vi "BSON_bytes_to_data_strict.vi"(7 "dataType":variant, 8 "error in (no error)":errorcluster, 11 "BSONbytes":u8[](array[numeric])) -> (0 "error out":errorcluster, 3 "result":variant)   [LabVIEW 2015, in "BSON_convertors_Library.lvlib"]
doc: "Converts the input byte stream into data fields and populates the input field with these values.\nNames, field types and their order must be the same in both structures"
uses:
  BSON_convertors_Library.lvlib
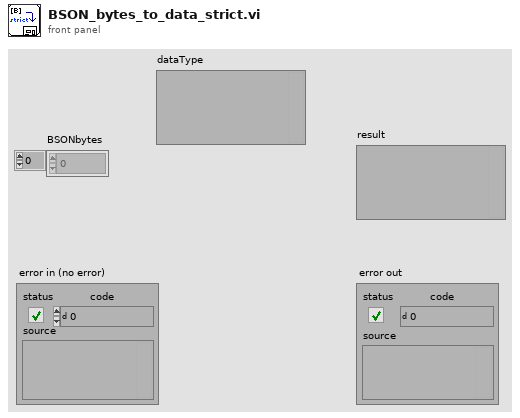
[diagram p1: front panel]
types:
  T1 = typedef "BSON_convertors_Library.lvlib/BSONelement.ctl" = cluster{"dataType":T2, "name":string, "value":variant}
  T2 = typedef "BSON_convertors_Library.lvlib/dataType.ctl" = enum8{"empty(terminator)", "double", "string", "document", "array", "binary", "Deprecated(Undefined)", "ObjectId", "boolean", "UTC datetime", "Null value", "cstring", "Deprecated(DBPointer)", "JavaScript", "Deprecated(Symbol)", "code_w_s", "int32", "uint64", "int64", "ext (decimal128)", "Min key", "Max key"}
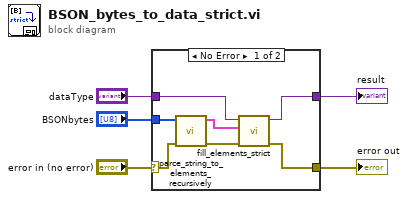
[diagram p0: block diagram]
diagram:
  n1 = case shown="No Error" "error in (no error)" {
    selector: "error in (no error)" -> [w11 w14]
    tunnel: "BSONbytes" -> [w12 _]
    tunnel: "dataType" -> [w10 w13]
    tunnel: [w6 w14] -> w2
    tunnel: [w7 w13] -> w1
    frame No Error {
      n2 = call "parce_string_to_elements_recursively.vi"("error in (no error)"=w11, "BSONdoc"=w12) -> ("error out"=w9:errorcluster, "arrayOfElements"=w8:T1[])  [unwired: 8 in]
      n3 = call "fill_elements_strict.vi"("error in (no error)"=w9, "arrayOfElements"=w8, "dataType in"=w10) -> ("error out"=w6:errorcluster, "dataType out"=w7:variant)  [unwired: 7 in]
    }
    frame Error {
    }
  }
  "result" <- w1
  "error out" <- w2
